vi "Write device and Session.vi"(8 "error in (no error)":errorcluster, 9 "device":refnum<k21>, 10 "session":refnum<k21>, 11 "SLSC Switch in":refnum<class "SLSC Switch.lvclass">) -> (0 "error out":errorcluster, 3 "SLSC Switch out":refnum<class "SLSC Switch.lvclass">)   [LabVIEW 2015, in "SLSC Switch.lvclass"]
uses:
  SLSC Switch.lvclass
  SLSC Switch.lvclass/SLSC Switch.ctl
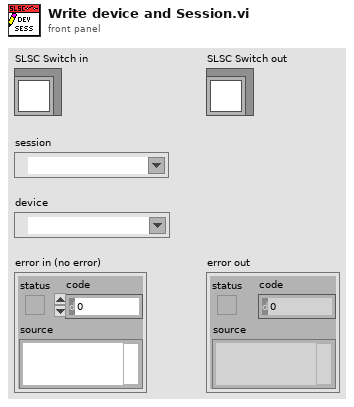
[diagram p1: front panel]
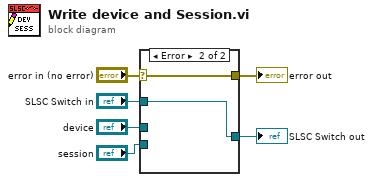
[diagram p0: block diagram]
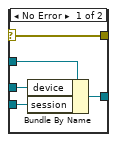
[diagram p2: hidden frame]
diagram:
  n1 = case shown="Error" "error in (no error)" {
    selector: "error in (no error)" -> [w11 w12]
    tunnel: [w11 w12] -> w5
    tunnel: [w9 w13] -> w3
    tunnel: "SLSC Switch in" -> [w10 w13]
    tunnel: "device" -> [w8 _]
    tunnel: "session" -> [w7 _]
    frame No Error {
      n2 = Bundle By Name(cluster=w10, "device"=w8, "session"=w7) -> (w9:refnum<class "SLSC Switch.lvclass">)
    }
    frame Error {
    }
  }
  "error out" <- w5
  "SLSC Switch out" <- w3
